vi "New sequence.vi"(8 "error in (no error)":errorcluster, 10 "Schedule":refnum<class "Schedule.lvclass">) -> (0 "error out":errorcluster, 3 "Run Block out":refnum<class "Run Block.lvclass">)   [LabVIEW 2020, in "TALOS.lvlib" / "Run Utilities.lvlib" / "Run Block.lvclass"]
doc: "Parses new schedule, and clears current RUN and skipped RUNs"
uses:
  Run Block.lvclass
  Schedule/Schedule.lvclass
  Run Instance/Run Instance.lvclass
  Run Block.lvclass/Run Block.ctl
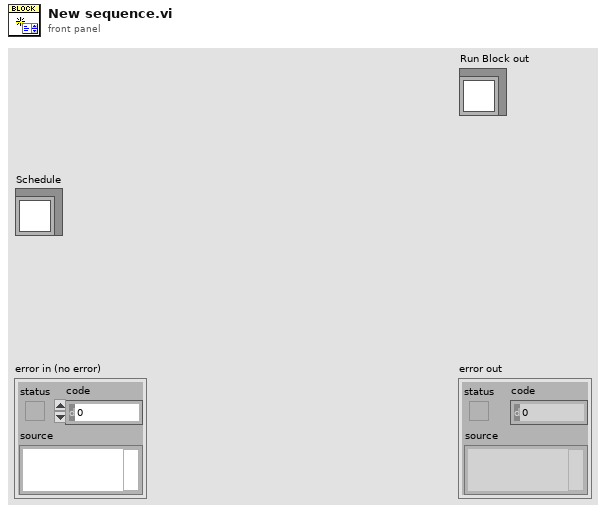
[diagram p1: front panel]
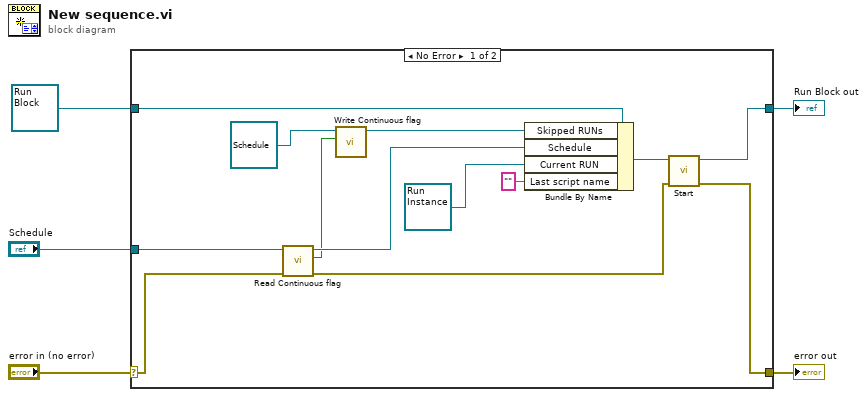
[diagram p0: block diagram]
diagram:
  n1 = case shown="No Error" "error in (no error)" {
    selector: "error in (no error)" -> [w16 w20]
    tunnel: [w6 w20] -> w4
    tunnel: [w8 w19] -> w2
    tunnel: refnum<class "Run Block.lvclass"> refnum ("Run Block in") -> [w15 w19]
    tunnel: "Schedule" -> [w17 _]
    frame No Error {
      n2 = call-dynamic "Read Continuous flag.vi"("error in (no error)"=w16, "Schedule in"=w17) -> ("error out"=w7:errorcluster, "Continuous flag"=w10:bool, "Schedule out"=w13:refnum<class "Schedule.lvclass">)  [unwired: 7 in]
      n3 = call-dynamic "Write Continuous flag.vi"("Continuous flag"=w10, "Schedule in"=refnum<class "Schedule.lvclass"> refnum ("Skipped RUNs")) -> ("Schedule out"=w14:refnum<class "Schedule.lvclass">)  [unwired: 8 in, 1 out]
      n4 = Bundle By Name(cluster=w15, "Skipped RUNs"=w14, "Schedule"=w13, "Current RUN"=refnum<class "Run Instance.lvclass"> refnum, "Last script name"="") -> (w9:refnum<class "Run Block.lvclass">)
      n5 = call-dynamic "Start.vi"("error in (no error)"=w7, "Run Block in"=w9) -> ("error out"=w6:errorcluster, "Run Block out"=w8:refnum<class "Run Block.lvclass">)  [unwired: 8 in]
    }
    frame Error {
    }
  }
  "error out" <- w4
  "Run Block out" <- w2
